vi "Main_FFT.vi"() -> ()   [LabVIEW 2026]
doc: "This template is for the Queued Message Handler design pattern.\n\nThe Event Handling Loop generates messages based on user interface actions.\n\nThe Message Handling Loop processes messages generated by the Event Handling Loop, or by other messages. The messages are string values, so new messages can be added easily to the Message Cases case structure in the Message Handling Loop. Each message cluster can also provide an optional value for Message Data, which is a variant that can be converted to whatever message-specific data is required."
uses:
  SubVIs/Controls/PCO_Config.ctl
  SubVIs/Controls/UI Data.ctl
  <instrlib>/PCO_SDK/File Group 0/vi.lib/Excelitas PCO GmbH/pco.labview/camera/Camera.lvclass
  SubVIs/Controls/TypeDef_FGV.ctl
  SubVIs/QMH/Message Queue/Enqueue Message (Single).vi
  SubVIs/QMH/Message Queue/Message Queue.lvlib
  SubVIs/QMH/User Event - Stop/User Event - Stop.lvlib
  <instrlib>/PCO_SDK/File Group 0/vi.lib/Excelitas PCO GmbH/pco.labview/pco.sdk/TimingControl/TimingControl.lvlib
panel:
  in  "# of frames":u16
  in  "SavePath":path
  out "FFT":dbl[][](graph)
  out "Graphe d'intensité":u16[][](graph)
  in  "Binning for FFT":u16(ring)=8 items=["1x1"=1, "2x2"=2, "4x4"=4, "8x8"=8]
  in  "Stop live":bool
  in  "FFT?":bool=TRUE
  in  "Grab":bool
  in  "Live":bool
  in  "PCO_Config":T1={"Exposure time (s)"=0.1, "TriggerMode"=0, "ROI X0"=1, "ROI Y0"=1, "ROI X1"=2048, "ROI Y1"=2048, "Binning"=1} {"TriggerMode" items=["auto sequence", "software trigger", "external exposure start", "external exposure control"]}
  out "Current task":string="\"Exit\" button pressed"
  in  "Exit":bool
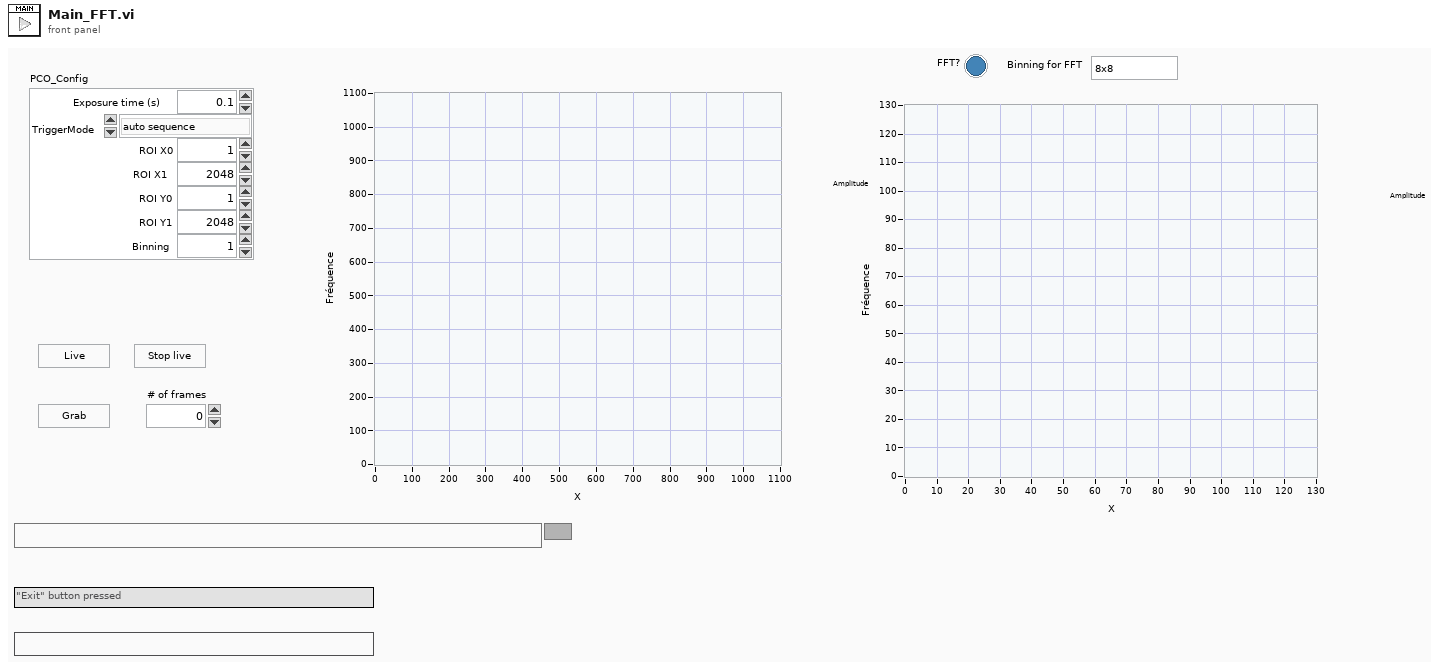
[diagram p1: front panel]
types:
  T1 = typedef "PCO_Config.ctl" = cluster{"Exposure time (s)":dbl, "TriggerMode":u16, "ROI X0":u16, "ROI Y0":u16, "ROI X1":u16, "ROI Y1":u16, "Binning":u8}
  T2 = typedef "UI Data.ctl" = cluster{"Data Display Ref":refnum<vi>, "Exit Button Ref":refnum<vi>, "Message":string}
  T3 = typedef "Message Queue.lvlib/All Message Queues.ctl" = cluster{"UI":refnum<queue>, "Camera loop":refnum<queue>, "Display loop":refnum<queue>}
  T4 = typedef "TypeDef_FGV.ctl" = enum16{"Initialize", "Write", "Read"}
  T5 = typedef "Camera.lvclass/binning.ctl" = cluster{"vert":u16, "horz":u16, "mode":u16}
  T6 = cluster{"exposure_time_s":dbl, "delay_time_s":dbl, "roi":cluster{"x0":u64, "y0":u64, "x1":u64, "y1":u64}, "timestamp_mode":u16, "pixelrate":u32, "trigger_mode":u16, "acquire_mode":u16, "metadata_mode":u16, "noisefilter_mode":u16, "pixel_format":u32, "binning":T5, "auto_exposure":cluster{"region":u16, "min_exposure_s":dbl, "max_exposure_s":dbl}}
  T7 = cluster{"wSignalNum":u16, "wEnabled":u16, "wType":u16, "wPolarity":u16, "wFilterSetting":u16, "wSelected":u16, "dwParameter":u32[], "dwSignalFunctionality":u32[]}
  T8 = cluster{"wVersion":u16, "dwIMAGE_COUNTER":u32, "dwIMAGE_TIME_US":u32, "lvTimestamp":timestamp, "bIMAGE_TIME_STATUS":u8, "wEXPOSURE_TIME_BASE":u16, "dwEXPOSURE_TIME":u32, "dwFRAMERATE_MILLIHZ":u32, "sSENSOR_TEMPERATURE":i16, "wIMAGE_SIZE_X":u16, "wIMAGE_SIZE_Y":u16, "bBINNING_X":u8, "bBINNING_Y":u8, "dwSENSOR_READOUT_FREQUENCY":u32, "wSENSOR_CONV_FACTOR":u16, "dwCAMERA_SERIAL_NO":u32, "wCAMERA_TYPE":u16, "bBIT_RESOLUTION":u8, "bSYNC_STATUS":u8, "wDARK_OFFSET":u16, "bTRIGGER_MODE":u8, "bDOUBLE_IMAGE_MODE":u8, "bCAMERA_SYNC_MODE":u8, "bIMAGE_TYPE":u8, "wCOLOR_PATTERN":u16, "wCAMERA_SUBTYPE":u16, "dwEVENT_NUMBER":u32, "wIMAGE_SIZE_X_Offset":u16, "wIMAGE_SIZE_Y_Offset":u16, "bREADOUT_MODE":u8}[]
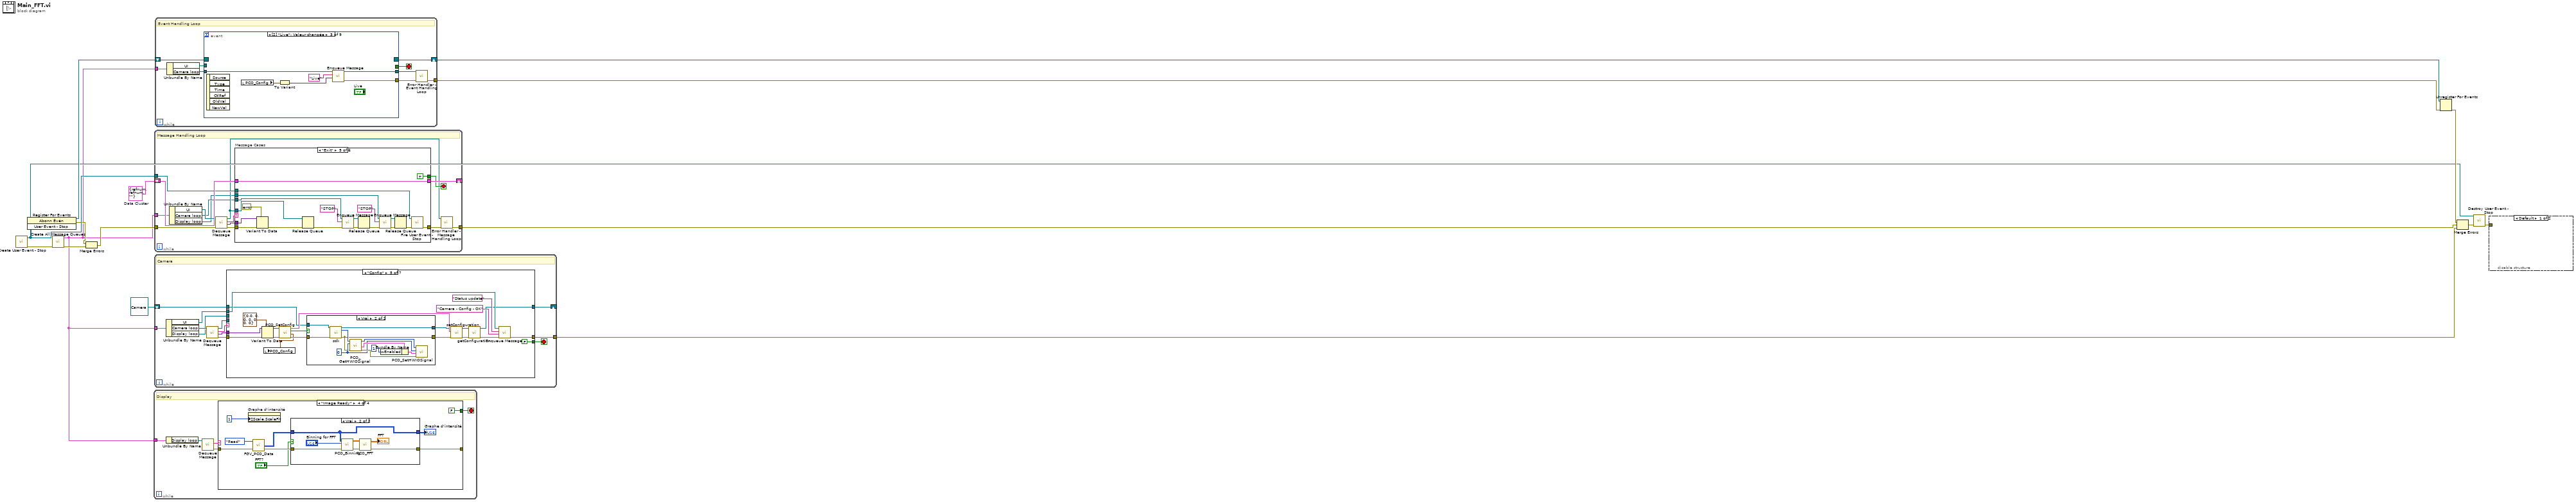
[diagram p0: block diagram]
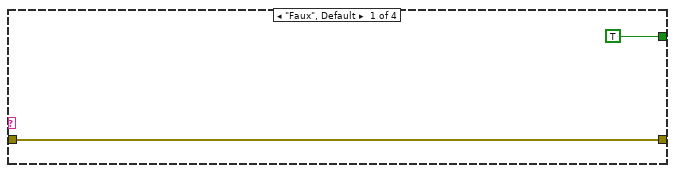
[diagram p2: hidden frame]
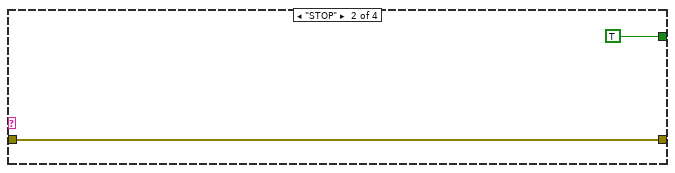
[diagram p3: hidden frame]
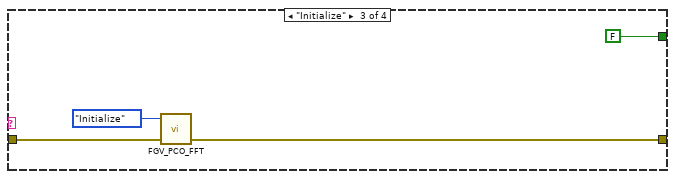
[diagram p4: hidden frame]
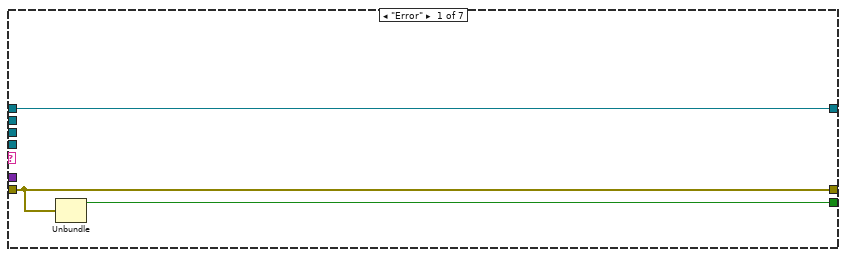
[diagram p6: hidden frame]
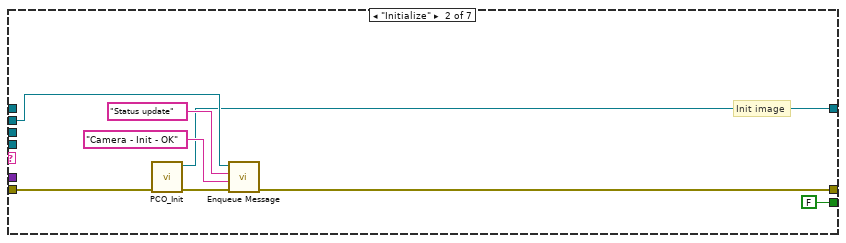
[diagram p7: hidden frame]
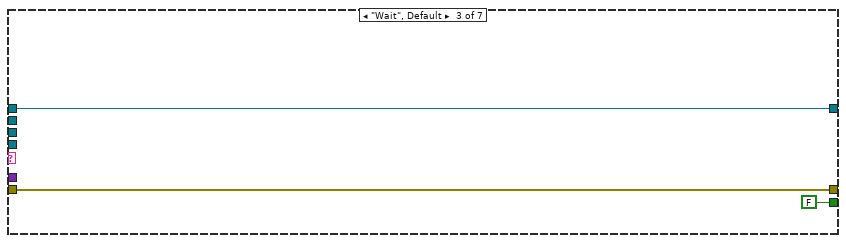
[diagram p8: hidden frame]
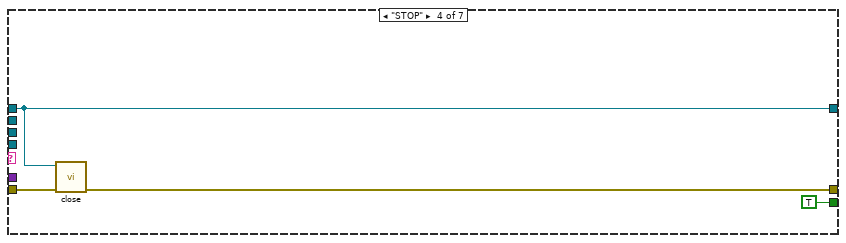
[diagram p9: hidden frame]
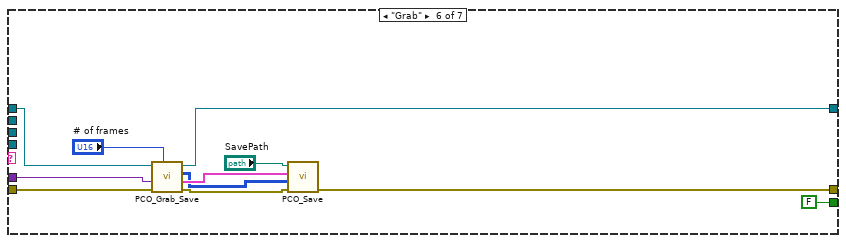
[diagram p11: hidden frame]
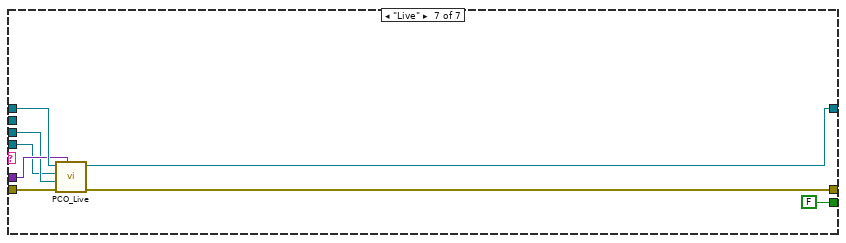
[diagram p12: hidden frame]
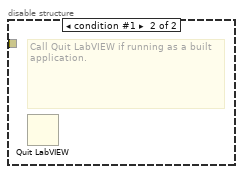
[diagram p13: hidden frame]
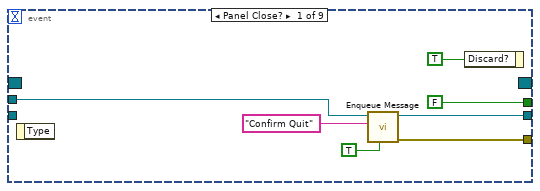
[diagram p14: hidden frame]
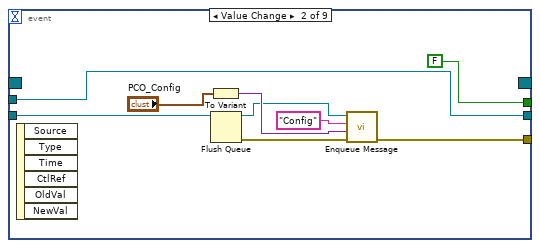
[diagram p15: hidden frame]
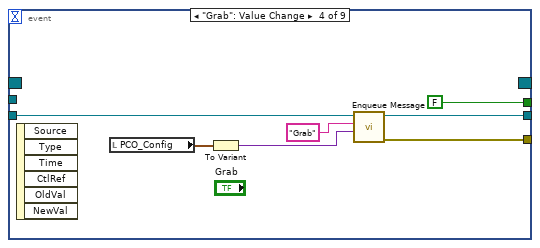
[diagram p16: hidden frame]
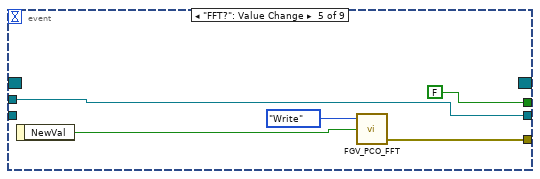
[diagram p17: hidden frame]
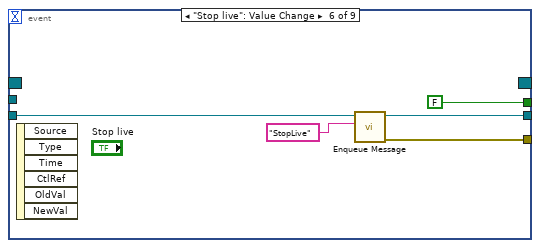
[diagram p18: hidden frame]
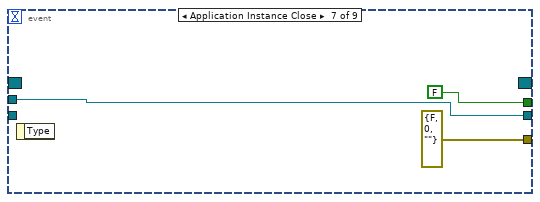
[diagram p19: hidden frame]
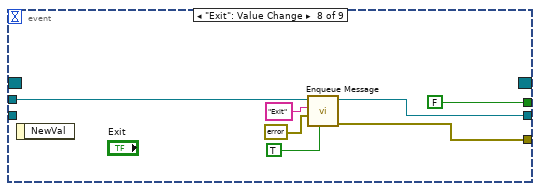
[diagram p20: hidden frame]
diagram:
  w4 = T2 {"Data Display Ref"=refnum, "Exit Button Ref"=refnum, "Message"=""}  # Data Cluster
  n1 = call "Create User Event - Stop.vi"() -> ("error out"=w14:errorcluster, "User Event - Stop"=w7:refnum<user-event>)  [unwired: 10 in]
  n2 = register-events(w7) -> (reference out=w8:refnum<event-registration>, error out=w5:errorcluster)  [unwired: 2 in]
  n3 = call "Create All Message Queues.vi"("error in (no error)"=w14) -> ("error out"=w16:errorcluster, "Message Queues out"=w2:T3)  [unwired: 9 in]
  n4 = Merge Errors(w5, w16) -> (w6:errorcluster)
  n5 = while {
    tunnel: w2 -> [w21]
    stop <- w17 stop-if-true
    # "Display"
    n6 = Unbundle By Name(w21) -> ("Display loop"=w20:refnum<queue>)
    n7 = call "Dequeue Message.vi"("Message Queue"=w20) -> ("error out"=w18:errorcluster, "Message"=w19:string)  [unwired: 7 in, 2 out]
    n8 = case shown="\"Image Ready\"" w19 {
      tunnel: w18 -> [w23 w24 w28 w37]
      tunnel: [w23 w24 w27 w31] -> _
      tunnel: [TRUE TRUE FALSE FALSE] -> w17
      frame "Faux", Default {
      }
      frame "STOP" {
      }
      frame "Initialize" {
        n9 = call "FGV_PCO_FFT.vi"("error in"=w28, "Action"=TypeDef_FGV."Initialize") -> ("error out"=w27:errorcluster)  [unwired: 2 in, 1 out]
      }
      frame "Image Ready" {
        n10 = property on="Graphe d'intensité" class="GraphInt (strict)"("ZScale.ScaleFit"=u8 1 ("Échelle des Z.Ajuster l'échelle")) -> ()  [unwired: 2 in, 2 out]
        n11 = call "FGV_PCO_Data.vi"("error in"=w37, "Action"=TypeDef_FGV."Read") -> ("error out"=w35:errorcluster, "Data"=w34:u16[][])  [unwired: 2 in]
        n12 = case shown="Vrai" "FFT?" {
          tunnel: [w40 w41] -> w31
          tunnel: w35 -> [w40 w47]
          tunnel: w34 -> [w39 w44]
          tunnel: [w39 w44] -> w32
          frame False {
          }
          frame True {
            n13 = call "PCO_Binning.vi"("error in"=w47, "Binning"="Binning for FFT", "Data"=w44) -> ("error out"=w46:errorcluster, "Data bin"=w45:dbl[][])  [unwired: 7 in]
            n14 = call "PCO_FFT.vi"("error in (no error)"=w46, "Data"=w45) -> ("error out"=w41:errorcluster, "FFT"=→"FFT":dbl[][])  [unwired: 8 in]
          }
        }
        "Graphe d'intensité" <- w32
      }
    }
  }
  n15 = while {
    tunnel: [w55] -> w3
    tunnel: w2 -> [w54]
    shift-right: [w52] -> _
    shift-left: refnum<class "Camera.lvclass"> refnum ("Camera out") -> [w51]
    stop <- w56 stop-if-true
    # "Camera"
    n16 = Unbundle By Name(w54) -> ("UI"=w53:refnum<queue>, "Camera loop"=w50:refnum<queue>, "Display loop"=w49:refnum<queue>)
    n17 = call "Dequeue Message.vi"("Message Queue"=w50) -> ("error out"=w59:errorcluster, "Message Data"=w57:variant, "Message"=w58:string, "dup Message Queue"=w48:refnum<queue>)  [unwired: 7 in]
    n18 = case shown="\"Config\"" w58 {
      tunnel: w59 -> [w62 w66 w73 w76 w97 w119 w128]
      tunnel: w57 -> [_ _ _ _ w96 w118 w127]
      tunnel: w53 -> [_ w70 _ _ w91 _ _]
      tunnel: [w61 FALSE ("status") FALSE ("status") TRUE FALSE ("status") FALSE ("status") FALSE ("status")] -> w56
      tunnel: [w62 w64 w73 w75 w90 w112 w125] -> w55
      tunnel: w48 -> [_ _ _ _ _ _ w123]
      tunnel: [w60 w65 w72 w74 w86 w122 w124] -> w52
      tunnel: w51 -> [w60 _ w72 w74 w84 w117 w129]
      tunnel: w49 -> [_ _ _ _ _ _ w126]
      frame "Error" {
        n19 = Unbundle(w62) -> ("status"=w61:bool)  [unwired: 2 out]
      }
      frame "Initialize" {
        # "Init image"
        n20 = call "PCO_Init.vi"("entrée d'erreur (pas d'erreur)"=w66) -> ("sortie d'erreur"=w63:errorcluster, "Camera en sortie"=w65:refnum<class "Camera.lvclass">)  [unwired: 9 in]
        n21 = call-poly "Enqueue Message.vi"("error in (no error)"=w63, "Message Data"="Camera - Init - OK", "Message"="Status update", "Message Queue"=w70) -> ("error out"=w64:errorcluster)  [unwired: 6 in, 1 out]
      }
      frame "Wait", Default {
      }
      frame "STOP" {
        n22 = call-dynamic "close.vi"("error in (no error)"=w76, "Camera in"=w74) -> ("error out"=w75:errorcluster)  [unwired: 9 in]
      }
      frame "Config" {
        n23 = Variant To Data(error in=w97, type=T1 {"Exposure time (s)"=0.0, "TriggerMode"=0, "ROI X0"=0, "ROI Y0"=0, "ROI X1"=0, "ROI Y1"=0, "Binning"=0} ("PCO_Config"), Variant=w96) -> (data=w94:T1, error out=w81:errorcluster)
        n24 = call "PCO_SetConfig.vi"("error in"=w81, "PCO_Config"=w94) -> ("error out"=w80:errorcluster, "PCO_Config 2"=w78:T1, "Trigger externe?"=w82:bool, "configuration"=w93:T6)  [unwired: 6 in]
        n25 = local write "PCO_Config"(w78) -> ()
        n26 = case shown="Vrai" w82 {
          tunnel: w80 -> [w100 w104]
          tunnel: [w100 w103] -> w85
          tunnel: w84 -> [w99 w102]
          tunnel: [w99 w101] -> w83
          frame False {
          }
          frame True {
            w106 = u16 0 ("wSignalNum")
            n27 = call-dynamic "sdk.vi"("Camera in"=w102, "error in (no error)"=w104) -> ("Camera out"=w101:refnum<class "Camera.lvclass">, "sdk"=w107:u64, "error out"=w103:errorcluster)  [unwired: 11 in]
            n28 = call <instrlib>:"PCO_GetHWIOSignal.vi"("error in (no error)"=w103, "wSignalNum"=w106, "ph"=w107) -> ("error out"=w109:errorcluster, "strSignal"=w111:T7, "ph out"=w108:u64)  [unwired: 5 in, 1 out]
            n29 = Bundle By Name(cluster=w111, "wEnabled"=u16 1) -> (w110:T7)
            n30 = call <instrlib>:"PCO_SetHWIOSignal.vi"("error in (no error)"=w109, "strSignal"=w110, "wSignalNum"=w106, "ph"=w108) -> ()  [unwired: 5 in, 3 out]
          }
        }
        n31 = call-dynamic "setConfiguration.vi"("error in (no error)"=w85, "configuration"=w93, "Camera in"=w83) -> ("error out"=w79:errorcluster, "Camera out"=w87:refnum<class "Camera.lvclass">)  [unwired: 7 in]
        n32 = call-dynamic "getConfiguration.vi"("error in (no error)"=w79, "Camera in"=w87) -> ("error out"=w88:errorcluster, "Camera out"=w86:refnum<class "Camera.lvclass">)  [unwired: 7 in, 1 out]
        n33 = call-poly "Enqueue Message.vi"("error in (no error)"=w88, "Message Data"="Camera - Config - OK", "Message"="Status update", "Message Queue"=w91) -> ("error out"=w90:errorcluster)  [unwired: 6 in, 1 out]
      }
      frame "Grab" {
        n34 = call "PCO_Grab_Save.vi"("# of frames"="# of frames", "entrée d'erreur (pas d'erreur)"=w119, "Message Data"=w118, "Camera en entrée"=w117) -> ("sortie d'erreur"=w115:errorcluster, "meta_data_list"=w114:T8, "Raw data (U16)"=w113:u16[][][], "Camera en sortie"=w122:refnum<class "Camera.lvclass">)  [unwired: 4 in]
        n35 = call "PCO_Save.vi"("entrée d'erreur (pas d'erreur)"=w115, "raw_image_list (U16)"=w113, "meta_data_list"=w114, "SavePath"="SavePath") -> ("sortie d'erreur"=w112:errorcluster)  [unwired: 7 in]
      }
      frame "Live" {
        n36 = call "PCO_Live.vi"("Message Data"=w127, "entrée d'erreur (pas d'erreur)"=w128, "Display loop"=w126, "dup Message Queue"=w123, "Camera en entrée"=w129) -> ("sortie d'erreur"=w125:errorcluster, "Camera en sortie"=w124:refnum<class "Camera.lvclass">)  [unwired: 5 in]
      }
    }
  }
  n37 = while {
    shift-right: [w144] -> _
    shift-left: w4 -> [w145]
    tunnel: w7 -> [w142]
    tunnel: w6 -> [w141]
    tunnel: [w136] -> w15
    tunnel: w2 -> [w134]
    stop <- w143 stop-if-true
    # "Message Handling Loop"
    n38 = Unbundle By Name(w134) -> ("UI"=w133:refnum<queue>, "Camera loop"=w132:refnum<queue>, "Display loop"=w131:refnum<queue>)
    n39 = call "Dequeue Message.vi"("error in (no error)"=w141, "Message Queue"=w133) -> ("error out"=w140:errorcluster, "Message Data"=w138:variant, "Message"=w139:string, "dup Message Queue"=w137:refnum<queue>)  [unwired: 6 in]
    n40 = case "Message Cases" shown="\"Exit\"" w139 {
      tunnel: w137 -> [w148 _ _ w170 w184 _]
      tunnel: w140 -> [w153 w159 w166 w172 w185 w193]
      tunnel: [w154 w156 w161 w167 w180 w193] -> w135
      tunnel: w145 -> [w152 w160 w165 w171 w192 w194]
      tunnel: [w151 w160 w165 w171 w192 w194] -> w144
      tunnel: [_ _ _ _ TRUE _] -> w143
      tunnel: w138 -> [_ w158 w164 _ w188 _]
      tunnel: w142 -> [_ _ _ _ w190 _]
      tunnel: w132 -> [_ _ _ _ w183 _]
      tunnel: w131 -> [_ _ _ _ w173 _]
      frame "Initialize" {
        w146 = "Initial Message" ("Initial Message")
        n41 = control-ref of="Current task"() -> (w147:refnum<vi>)
        n42 = control-ref of="Exit"() -> (w150:refnum<vi>)
        n43 = Bundle By Name(cluster=w152, "Data Display Ref"=w147, "Exit Button Ref"=w150, "Message"=w146) -> (w151:T2)
        n44 = call-poly "Enqueue Message.vi"("error in (no error)"=w153, "Message Data"=w146, "Message"="Update Display", "Message Queue"=w148) -> ("error out"=w154:errorcluster)  [unwired: 6 in, 1 out]
      }
      frame "Update Display" {
        n45 = Variant To Data(error in=w159, type="", Variant=w158) -> (data=→"Current task":string, error out=w156:errorcluster)
      }
      frame "Error" {
        n46 = Variant To Data(error in=w166, type=errorcluster {"status"=FALSE, "code"=0, "source"=""} ("error constant"), Variant=w164) -> (data=w162:errorcluster, error out=w161:errorcluster)
        n47 = call <vilib>:"Simple Error Handler.vi"("error in (no error)"=w162) -> ()  [unwired: 4 in, 5 out]
      }
      frame "Confirm Quit" {
        n48 = call-poly "Enqueue Message.vi"("Priority Message? (F)"=TRUE, "error in (no error)"=w172, "Message"="Exit", "Message Queue"=w170) -> ("error out"=w167:errorcluster)  [unwired: 6 in, 1 out]
      }
      frame "Exit" {
        n49 = Variant To Data(error in=w185, type=errorcluster {"status"=FALSE, "code"=0, "source"=""} ("error constant"), Variant=w188) -> (error out=w181:errorcluster)  [unwired: 1 out]
        n50 = Release Queue(queue=w184, error in (no error)=w181) -> (error out=w179:errorcluster)  [unwired: 1 in, 2 out]
        n51 = call-poly "Enqueue Message.vi"("error in (no error)"=w179, "Message"="STOP", "Message Queue"=w183) -> ("error out"=w187:errorcluster, "dup Message Queue"=w186:refnum<queue>)  [unwired: 7 in]
        n52 = Release Queue(queue=w186, error in (no error)=w187) -> (error out=w175:errorcluster)  [unwired: 1 in, 2 out]
        n53 = call-poly "Enqueue Message.vi"("error in (no error)"=w175, "Message"="STOP", "Message Queue"=w173) -> ("error out"=w176:errorcluster, "dup Message Queue"=w177:refnum<queue>)  [unwired: 7 in]
        n54 = Release Queue(queue=w177, error in (no error)=w176) -> (error out=w174:errorcluster)  [unwired: 1 in, 2 out]
        n55 = call "Fire User Event - Stop.vi"("error in (no error)"=w174, "User Event - Stop"=w190) -> ("error out"=w180:errorcluster)  [unwired: 9 in]
      }
      frame Default {
      }
    }
    n56 = call "Error Handler - Message Handling Loop.vi"("error in (no error)"=w135, "Message Queue"=w137) -> ("dup error in"=w136:errorcluster)  [unwired: 8 in, 1 out]
  }
  n57 = while {
    shift-right: [w202] -> w11
    shift-left: w8 -> [w203]
    tunnel: [w198] -> w9
    tunnel: w2 -> [w195]
    stop <- w200 stop-if-true
    # "Event Handling Loop"
    n58 = Unbundle By Name(w195) -> ("UI"=w197:refnum<queue>, "Camera loop"=w196:refnum<queue>)
    n59 = event shown="[2] \"Live\": Valeur changée" {
      selector: w203 -> [_ _ _ _ _ _ _ _ _]
      dyn-events: [_ _ _ _ _ _ _ _ _] -> w202
      timeout: _ -> [_ _ _ _ _ _ _ _ _]
      tunnel: [FALSE ("Discard?") FALSE ("Discard?") _ FALSE ("Discard?") FALSE ("Discard?") FALSE ("Discard?") FALSE ("Discard?") FALSE ("Discard?") TRUE ("Discard?")] -> w200
      tunnel: w197 -> [w209 w219 _ _ w237 _ w245 w252 w256]
      tunnel: [w208 w215 w222 w229 w235 w240 errorcluster {"status"=FALSE, "code"=0, "source"=""} ("error out") w246 errorcluster {"status"=FALSE, "code"=0, "source"=""} ("error out")] -> w201
      tunnel: [w207 w219 w221 w230 w237 w239 w245 w251 w256] -> w199
      tunnel: w196 -> [_ w213 w220 w231 _ w241 _ _ _]
      event Panel Close? {
        n60 = event-data() -> ()  [unwired: 1 in, 1 out]
        n61 = call-poly "Enqueue Message.vi"("Priority Message? (F)"=TRUE, "Message"="Confirm Quit", "Message Queue"=w209) -> ("error out"=w208:errorcluster, "dup Message Queue"=w207:refnum<queue>)  [unwired: 7 in]
        n62 = event-data("Discard?"=TRUE) -> ()  [unwired: 1 in, 1 out]
      }
      event Value Change {
        n63 = event-data() -> ()  [unwired: 1 in, 6 out]
        n64 = To Variant(anything="PCO_Config") -> (Variant=w216:variant)
        n65 = Flush Queue(queue=w213) -> (queue out=w211:refnum<queue>, error out=w212:errorcluster)  [unwired: 1 in, 1 out]
        n66 = call-poly "Enqueue Message.vi"("error in (no error)"=w212, "Message Data"=w216, "Message"="Config", "Message Queue"=w211) -> ("error out"=w215:errorcluster)  [unwired: 6 in, 1 out]
      }
      event "Live": Value Change {
        n67 = event-data() -> ()  [unwired: 1 in, 6 out]
        n68 = local read "PCO_Config"() -> (w225:T1)
        n69 = To Variant(anything=w225) -> (Variant=w224:variant)
        n70 = call-poly "Enqueue Message.vi"("Message Data"=w224, "Message"="Live", "Message Queue"=w220) -> ("error out"=w222:errorcluster, "dup Message Queue"=w221:refnum<queue>)  [unwired: 7 in]
      }
      event "Grab": Value Change {
        n71 = event-data() -> ()  [unwired: 1 in, 6 out]
        n72 = local read "PCO_Config"() -> (w227:T1)
        n73 = To Variant(anything=w227) -> (Variant=w226:variant)
        n74 = call-poly "Enqueue Message.vi"("Message Data"=w226, "Message"="Grab", "Message Queue"=w231) -> ("error out"=w229:errorcluster, "dup Message Queue"=w230:refnum<queue>)  [unwired: 7 in]
      }
      event "FFT?": Value Change {
        n75 = event-data() -> ("NewVal"=w233:bool)  [unwired: 1 in]
        n76 = call "FGV_PCO_FFT.vi"("FFT?"=w233, "Action"=TypeDef_FGV."Write") -> ("error out"=w235:errorcluster)  [unwired: 2 in, 1 out]
      }
      event "Stop live": Value Change {
        n77 = event-data() -> ()  [unwired: 1 in, 6 out]
        n78 = call-poly "Enqueue Message.vi"("Message"="StopLive", "Message Queue"=w241) -> ("error out"=w240:errorcluster, "dup Message Queue"=w239:refnum<queue>)  [unwired: 8 in]
      }
      event Application Instance Close {
        n79 = event-data() -> ()  [unwired: 1 in, 1 out]
      }
      event "Exit": Value Change {
        n80 = event-data() -> ()  [unwired: 1 in, 1 out]
        n81 = call-poly "Enqueue Message.vi"("Priority Message? (F)"=TRUE, "Message Data"=errorcluster {"status"=FALSE, "code"=0, "source"=""} ("error constant"), "Message"="Exit", "Message Queue"=w252) -> ("error out"=w246:errorcluster, "dup Message Queue"=w251:refnum<queue>)  [unwired: 6 in]
      }
      event User Event {
        n82 = event-data() -> ()  [unwired: 1 in, 1 out]
        n83 = local write "Current task"("\"Exit\" button pressed" ("VI Stopped")) -> ()
      }
    }
    n84 = call "Error Handler - Event Handling Loop.vi"("error in (no error)"=w201, "Message Queue"=w199) -> ("dup error in"=w198:errorcluster)  [unwired: 8 in, 1 out]
  }
  n85 = Unregister For Events(event registration refnum=w11, error in=w9) -> (error out=w12:errorcluster)
  n86 = Merge Errors(w12, w15, w3) -> (w13:errorcluster)
  n87 = call "Destroy User Event - Stop.vi"("error in (no error)"=w13, "User Event - Stop"=w7) -> ("error out"=w10:errorcluster)  [unwired: 9 in]
  n88 = disable-structure shown="Default" {
    disable-tunnel: w10 -> [_ _]
    frame condition #0 (active) {
    }
    frame condition #1 {
      # "Call Quit LabVIEW if running as a built application."
      n89 = Quit LabVIEW() -> ()  [unwired: 1 in]
    }
  }
